vi "Read Optical Smoothing Level.vi"(8 "error in (no error)":errorcluster, 11 "StellarNetSpectrometer in":refnum<class "StellarNetSpectrometer.lvclass">) -> (0 "error out":errorcluster, 2 "Optical Smoothing Level":i32 min=0 max=4 step=1, 3 "StellarNetSpectrometer out":refnum<class "StellarNetSpectrometer.lvclass">)   [LabVIEW 2013, in "StellarNetSpectrometer.lvclass"]
uses:
  StellarNetSpectrometer.lvclass
  StellarNetSpectrometer.lvclass/StellarNetSpectrometer.ctl
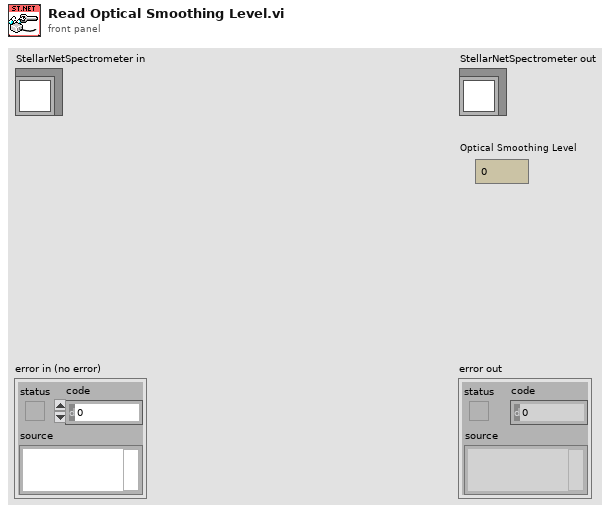
[diagram p1: front panel]
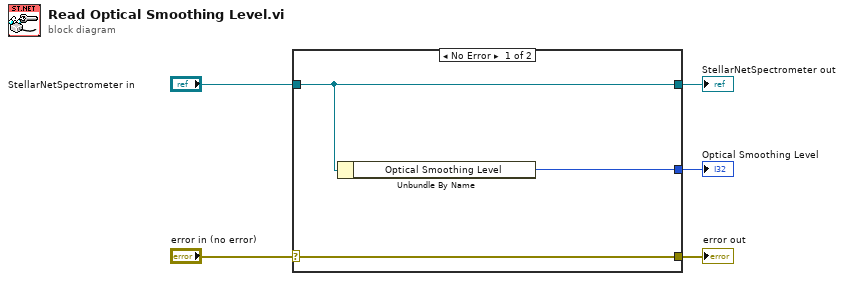
[diagram p0: block diagram]
diagram:
  n1 = case shown="No Error" "error in (no error)" {
    selector: "error in (no error)" -> [w8 w9]
    tunnel: [w8 w9] -> w4
    tunnel: [w7 w10] -> w2
    tunnel: "StellarNetSpectrometer in" -> [w7 w10]
    tunnel: [w6 _] -> w1
    frame No Error {
      n2 = Unbundle By Name(w7) -> ("Optical Smoothing Level"=w6:i32)
    }
    frame Error {
    }
  }
  "error out" <- w4
  "StellarNetSpectrometer out" <- w2
  "Optical Smoothing Level" <- w1
